vi "Teleop.vi"(10 "Match Info":T1={"Autonomous Elapsed Seconds"=0.0, "TeleOp Elapsed Seconds"=0.0, "Disabled Elapsed Seconds"=0.0, "Visited Autonomous"=FALSE, "Visited TeleOp"=FALSE, "Visited Disabled"=FALSE, "Autonomous Settings"={"Autonomous Style"=enum."Independent", "VI Refnum"=refnum}}, 11 "Call Context":T2) -> ()   [LabVIEW 2016]
doc: "This VI is called for each TeleOp packet received from the DS where the robot is not disabled. It is often used to read from the joysticks and update I/O or to update setpoints for timed control loops. It should complete and return within 20 milliseconds or it may miss DS packets."
uses:
  <vilib>/Rock Robotics/WPI/DriverStation/WPI_DriverStationDerivedRobotMode.ctl
  <vilib>/Rock Robotics/WPI/DriverStation/WPI_DriverStationMatch Info.ctl
  <vilib>/Rock Robotics/WPI/Relay/WPI_RelayValue.ctl
  <vilib>/Rock Robotics/WPI/Solenoid/WPI_SolenoidValue.ctl
  <vilib>/Rock Robotics/WPI/Utilities/WPI_GetSetVariantRefNum.vi
  <vilib>/Rock Robotics/Network Tables/NT Write Boolean Array.vi
  <vilib>/Rock Robotics/Network Tables/NT Write Numeric Array.vi
  <vilib>/Rock Robotics/Network Tables/NT Read Boolean.vi
  <vilib>/Rock Robotics/Network Tables/NT Read Number.vi
  <vilib>/Rock Robotics/WPI/RobotDrive/WPI_RobotDriveMecanumDrive_Cartesian.vi
  <vilib>/Rock Robotics/WPI/Solenoid/WPI_SolenoidSetEnum.vi
panel:
  out "Joystick Button 12":bool
  out "Joystick Button 8":bool
  in  "Test Switch 1":bool
  in  "Test Switch 3":bool
  in  "Test Switch 2":bool
  out "Ctl State 3":dbl
  out "Joystick Button 6":bool
  out "Joystick Button 4":bool
  out "Ctl State 2":dbl
  out "Joystick Button 3":bool
  out "Joystick Button 5":bool
  out "Ctl State":dbl
  out "Joystick Button 11":bool
  out "Joystick Button 7":bool
  out "Joystick Test Y":dbl
  out "Sample Slider 0":dbl(slide) scale=0.0..5.0
  out "Sample Boolean 1":bool
  out "Sample Boolean 0":bool
  # "Rope Collector"
  # "Rope Collector"
  # "Gear Arm"
  # "Gear Gripper"
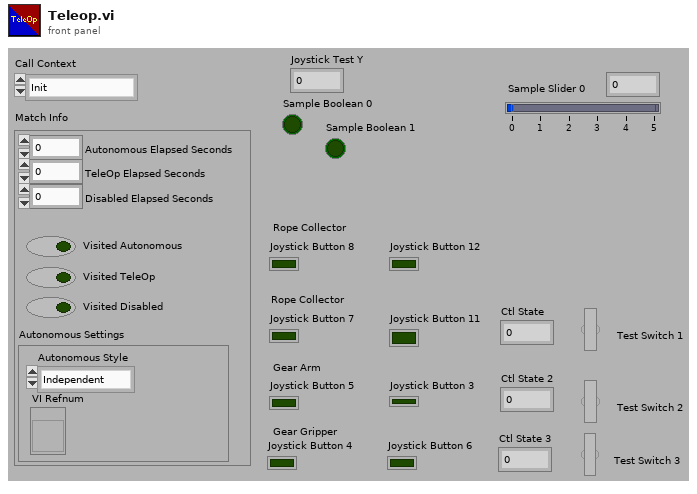
[diagram p1: front panel]
types:
  T1 = typedef "WPI_DriverStationMatch Info.ctl" = cluster{"Autonomous Elapsed Seconds":dbl, "TeleOp Elapsed Seconds":dbl, "Disabled Elapsed Seconds":dbl, "Visited Autonomous":bool, "Visited TeleOp":bool, "Visited Disabled":bool, "Autonomous Settings":cluster{"Autonomous Style":enum16{"Iterative", "Independent"}, "VI Refnum":refnum<vi>}}
  T2 = typedef "WPI_DriverStationDerivedRobotMode.ctl" = enum16{"Init", "Execute", "Stop"}
  T3 = typedef "WPI_RelayValue.ctl" = enum16{"Off", "On", "Forward", "Reverse"}
  T4 = typedef "WPI_CompressorDevRef.ctl" = cluster{"DevStatus":errorcluster, "Pneumatics Control Module":u8}
  T5 = typedef "WPI_RobotDriveDevRef.ctl" = cluster{"DevStatus":errorcluster, "Motors[]":T6[], "Square Inputs":bool, "Max Output":dbl}
  T6 = typedef "WPI_MotorControlDeviceRef.ctl" = cluster{"DeviceStatus":errorcluster, "Type":T7, "PWM":cluster{"PWM Channel":T8, "DeadBand":T9}, "CAN":cluster{"Device Number":u8, "SetOutput VI Ref":variant, "GetOutput VI Ref":variant, "Enable VI Ref":variant, "Disable VI Ref":variant, "Data":variant}, "Invert":bool}
  T7 = typedef "WPI_MotorControlType.ctl" = enum16{"PWM", "CAN"}
  T8 = typedef "FPGA_DIOPWMChannel.ctl" = enum8{"PWM 0", "PWM 1", "PWM 2", "PWM 3", "PWM 4", "PWM 5", "PWM 6", "PWM 7", "PWM 8", "PWM 9", "PWM MXP 0", "PWM MXP 1", "PWM MXP 2", "PWM MXP 3", "PWM MXP 4", "PWM MXP 5", "PWM MXP 6", "PWM MXP 7", "PWM MXP 8", "PWM MXP 9", "Invalid"}
  T9 = typedef "WPI_PWMDeadband.ctl" = cluster{"Name":string, "maxPositivePwm":i32, "minPositivePwm":i32, "centerPwm":i32, "maxNegativePwm":i32, "minNegativePwm":i32, "angularRange":u16}
  T10 = typedef "WPI_JoystickDevRef.ctl" = cluster{"Device":T11}
  T11 = typedef "WPI_JoystickDeviceEnum.ctl" = enum16{"USB 0", "USB 1", "USB 2", "USB 3", "USB 4", "USB 5"}
  T12 = cluster{"Buttons[0]":bool, "Buttons[1]":bool, "Buttons[2]":bool, "Buttons[3]":bool, "Buttons[4]":bool, "Buttons[5]":bool, "Buttons[6]":bool, "Buttons[7]":bool, "Buttons[8]":bool}
  T13 = cluster{"Axes[0]":dbl, "Axes[1]":dbl, "Axes[2]":dbl, "Axes[3]":dbl, "Axes[4]":dbl, "Axes[5]":dbl, "Axes[6]":dbl, "Axes[7]":dbl, "Axes[8]":dbl}
  T14 = typedef "WPI_RelayDevRef.ctl" = cluster{"DevStatus":errorcluster, "Relay Channel":T15, "Relay Direction":T16}
  T15 = typedef "FPGA_DIORelayChannel.ctl" = enum8{"Relay 0", "Relay 1", "Relay 2", "Relay 3", "Invalid"}
  T16 = typedef "WPI_RelayDirection.ctl" = enum16{"Both directions", "Forward only", "Reverse only"}
  T17 = typedef "WPI_SolenoidDevRef.ctl" = cluster{"DevStatus":errorcluster, "Pneumatics Control Module":u8, "Forward Solenoid Channel":T18, "Reverse Solenoid Channel":T18}
  T18 = typedef "WPI_SolenoidChannel.ctl" = enum8{"Solenoid 0", "Solenoid 1", "Solenoid 2", "Solenoid 3", "Solenoid 4", "Solenoid 5", "Solenoid 6", "Solenoid 7", "Invalid"}
  T19 = typedef "WPI_SolenoidValue.ctl" = enum16{"Off", "On", "Forward", "Reverse"}
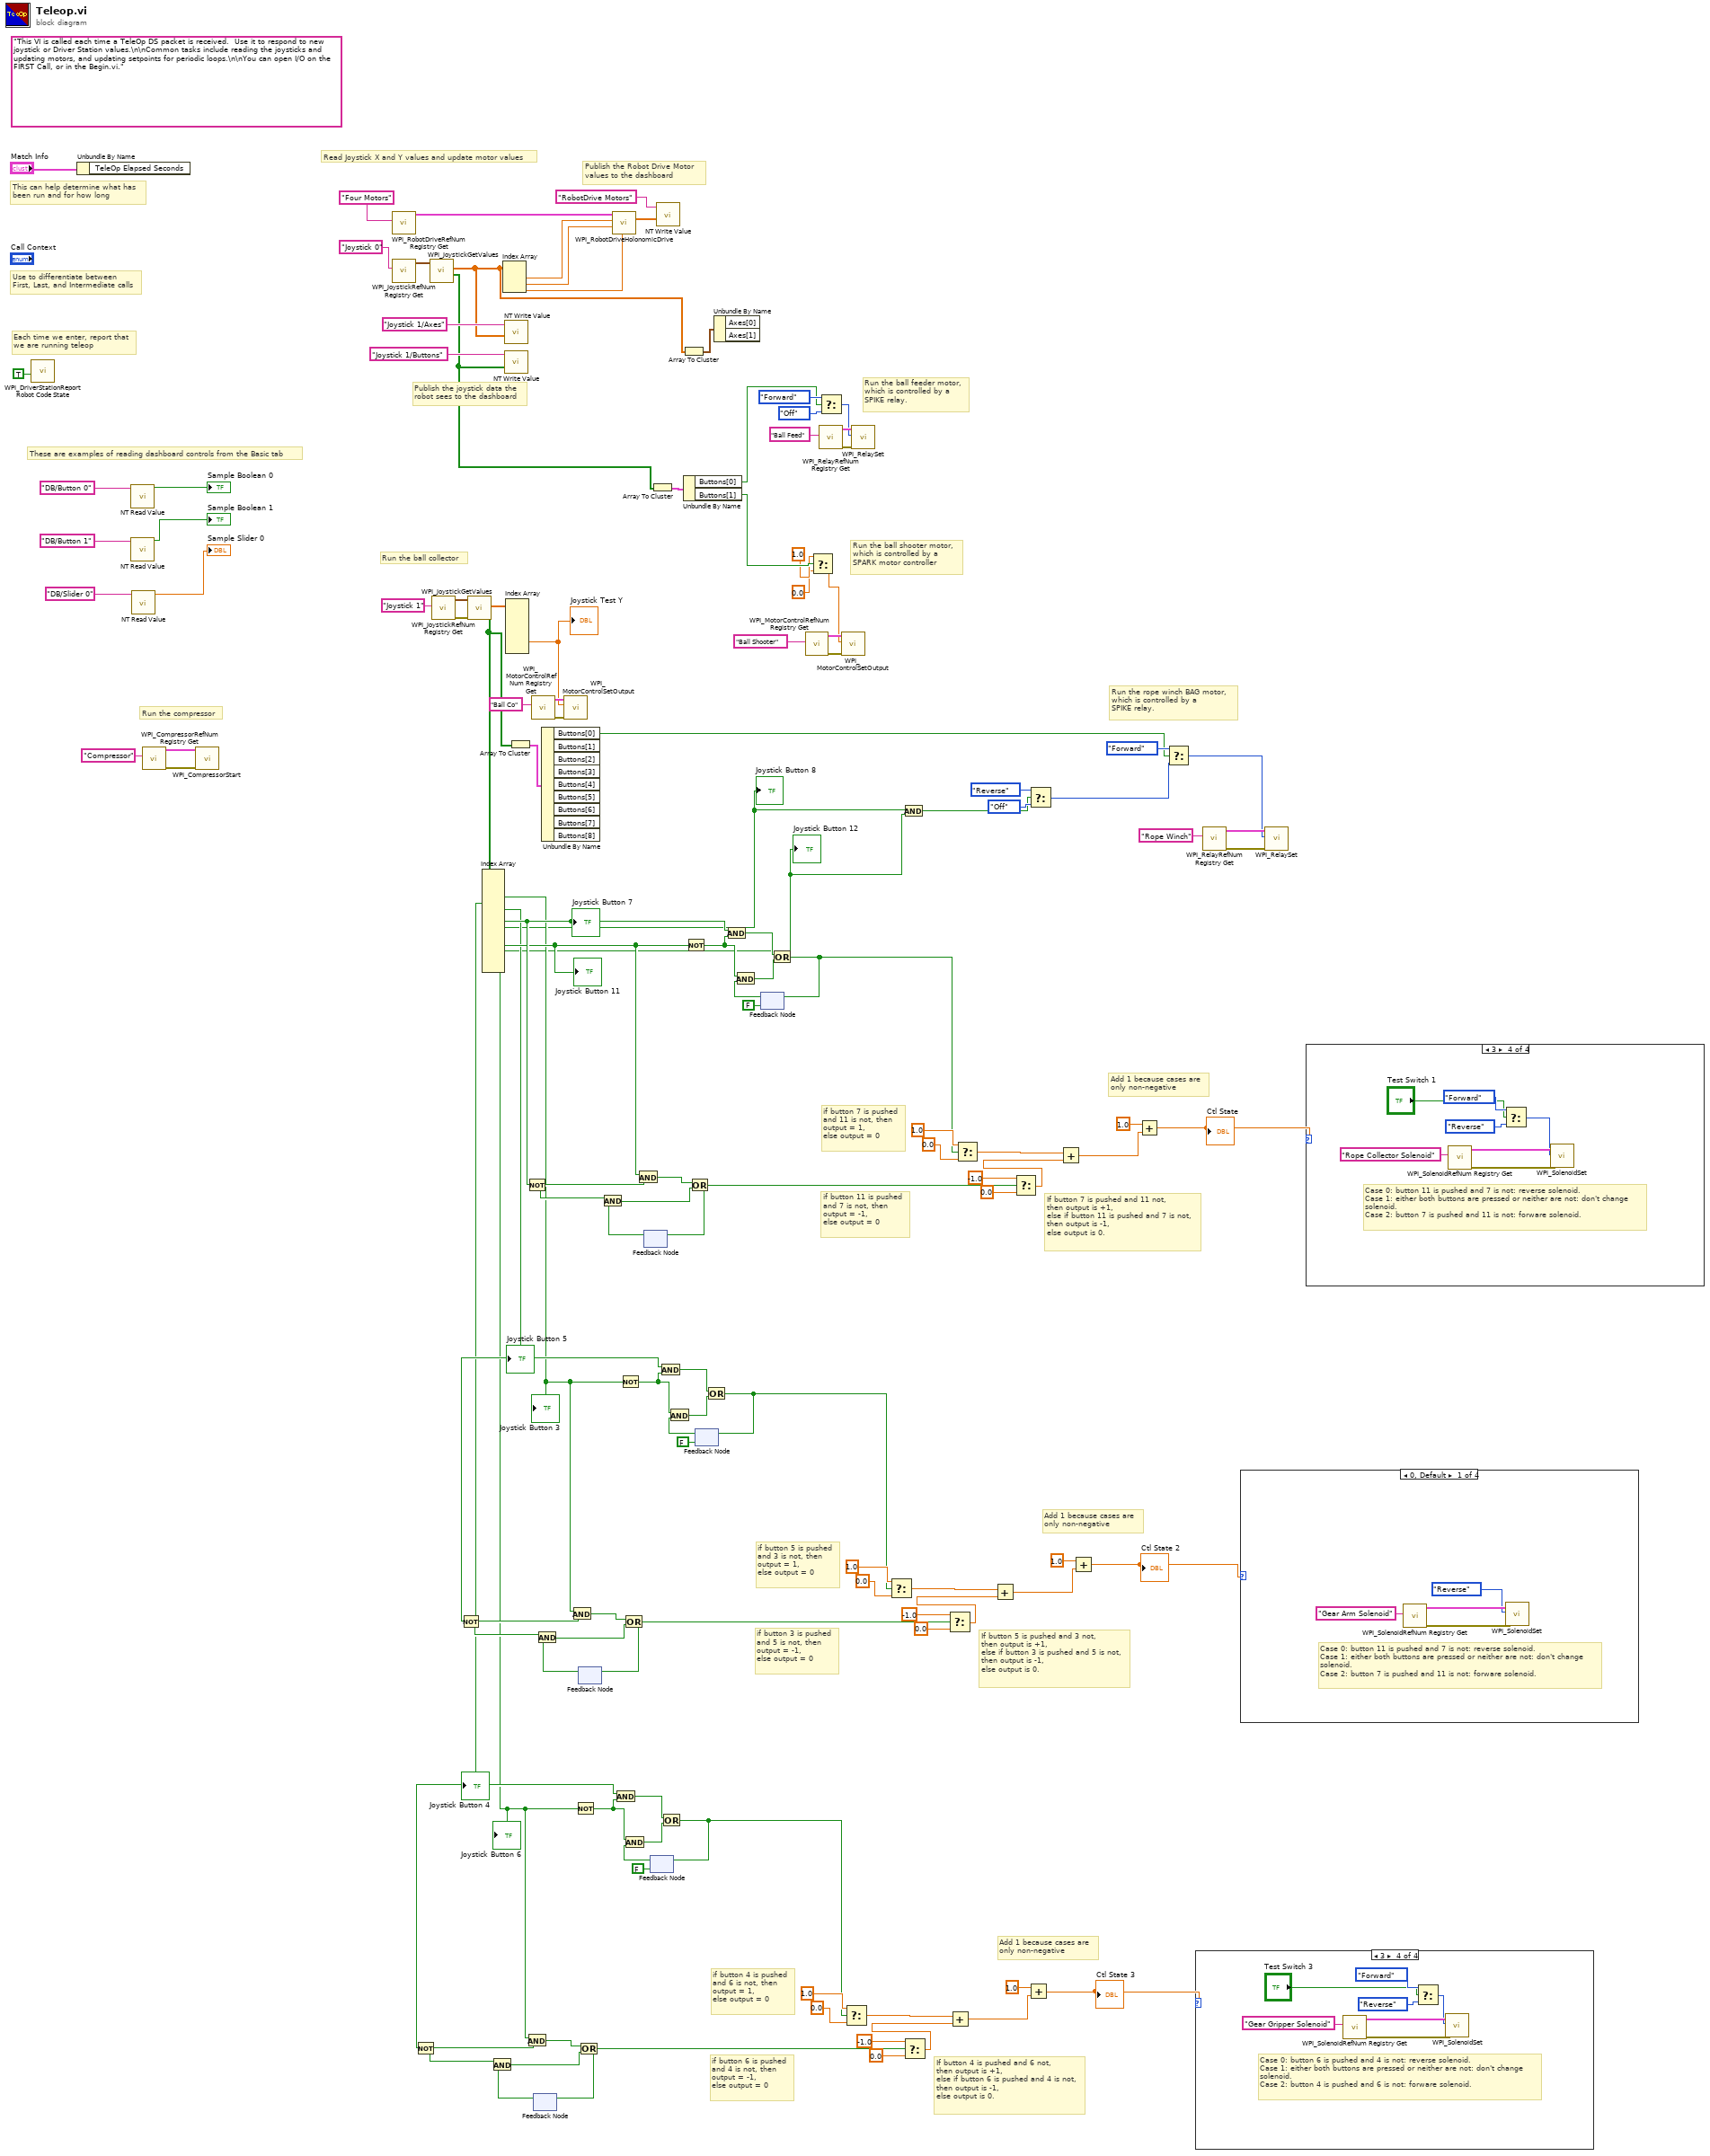
[diagram p0: block diagram]
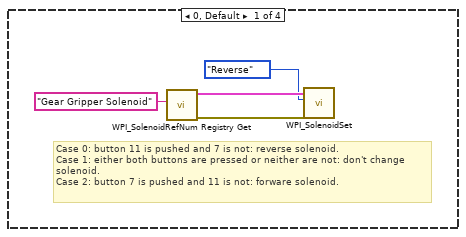
[diagram p2: hidden frame]
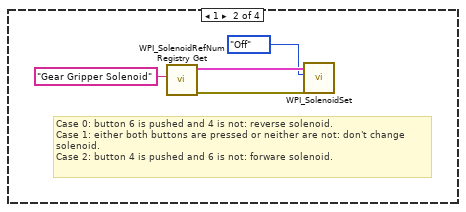
[diagram p3: hidden frame]
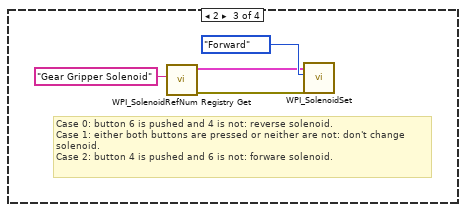
[diagram p4: hidden frame]
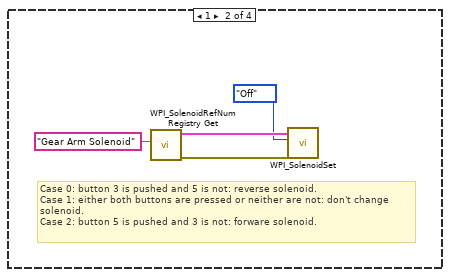
[diagram p5: hidden frame]
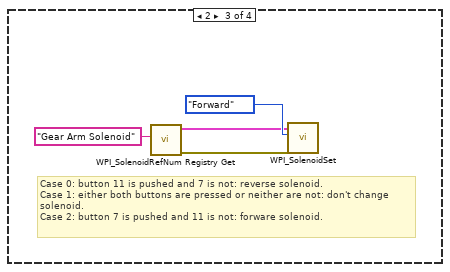
[diagram p6: hidden frame]
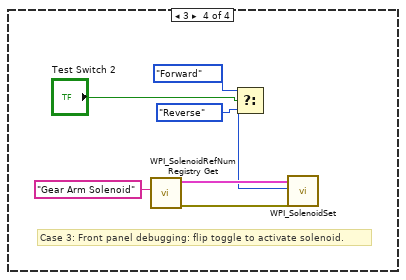
[diagram p7: hidden frame]
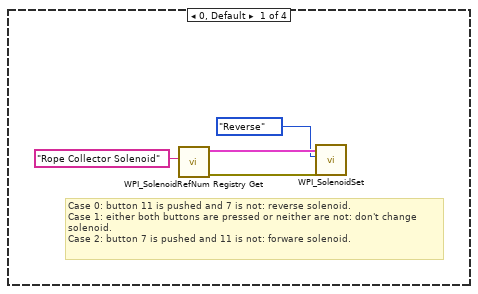
[diagram p8: hidden frame]
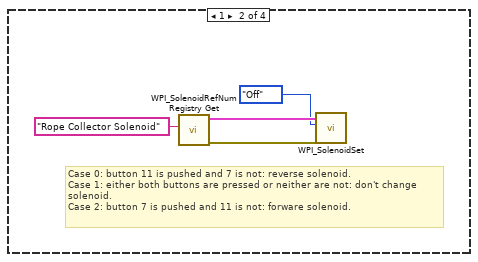
[diagram p9: hidden frame]
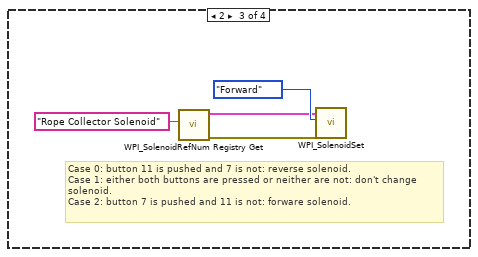
[diagram p10: hidden frame]
diagram:
  (unwired) "This VI is called each time a TeleOp DS packet is received.  Use it to respond to new joystick or Driver Station values.\n\nCommon tasks include reading the joysticks and updating motors, and updating setpoints for periodic loops.\n\nYou can open I/O on the FIRST Call, or in the Begin.vi."
  # "Add 1 because cases are \nonly non-negative"
  # "If button 4 is pushed and 6 not,\nthen output is +1,\nelse if button 6 is pushed and 4 is not,\nthen output is -1,\nelse output is 0."
  # "if button 6 is pushed\nand 4 is not, then\noutput = -1,\nelse output = 0"
  # "if button 4 is pushed\nand 6 is not, then\noutput = 1,\nelse output = 0"
  # "Add 1 because cases are \nonly non-negative"
  # "If button 5 is pushed and 3 not,\nthen output is +1,\nelse if button 3 is pushed and 5 is not,\nthen output is -1,\nelse output is 0."
  # "if button 3 is pushed\nand 5 is not, then\noutput = -1,\nelse output = 0"
  # "if button 5 is pushed\nand 3 is not, then\noutput = 1,\nelse output = 0"
  # "Add 1 because cases are \nonly non-negative"
  # "If button 7 is pushed and 11 not,\nthen output is +1,\nelse if button 11 is pushed and 7 is not,\nthen output is -1,\nelse output is 0."
  # "if button 11 is pushed\nand 7 is not, then\noutput = -1,\nelse output = 0"
  # "if button 7 is pushed\nand 11 is not, then\noutput = 1,\nelse output = 0"
  # "Run the compressor"
  # "Run the rope winch BAG motor,\nwhich is controlled by a \nSPIKE relay."
  # "Run the ball feeder motor,\nwhich is controlled by a \nSPIKE relay."
  # "Run the ball shooter motor,\nwhich is controlled by a \nSPARK motor controller"
  # "Run the ball collector"
  # "These are examples of reading dashboard controls from the Basic tab"
  # "Publish the Robot Drive Motor\nvalues to the dashboard"
  # "Publish the joystick data the\nrobot sees to the dashboard"
  # "Each time we enter, report that\nwe are running teleop"
  # "Use to differentiate between\nFirst, Last, and Intermediate calls"
  # "This can help determine what has\nbeen run and for how long"
  # "Read Joystick X and Y values and update motor values"
  n1 = call <vilib>:"WPI_DriverStationReport Robot Code State.vi"("TeleOp"=TRUE ("Autonomous")) -> ()  [unwired: 10 in, 1 out]
  n2 = Unbundle By Name("Match Info") -> ()  [unwired: 1 out]
  n3 = call-poly <vilib>:"NT Read Value.vi"("Name"="DB/Button 0" ("refnum name")) -> ("Boolean"=→"Sample Boolean 0":bool)  [unwired: 9 in, 1 out]
  n4 = call-poly <vilib>:"NT Read Value.vi"("Name"="DB/Button 1" ("refnum name")) -> ("Boolean"=→"Sample Boolean 1":bool)  [unwired: 9 in, 1 out]
  n5 = call-poly <vilib>:"NT Read Value.vi"("Name"="DB/Slider 0" ("refnum name")) -> ("Numeric"=→"Sample Slider 0":dbl)  [unwired: 9 in, 1 out]
  n6 = call <vilib>:"WPI_CompressorRefNum Registry Get.vi"("refnum name"="Compressor") -> ("error out"=w79:errorcluster, "CompressorDevRef"=w80:T4)  [unwired: 9 in]
  n7 = call <vilib>:"WPI_CompressorStart.vi"("error in (no error)"=w79, "CompressorDevRef"=w80) -> ()  [unwired: 8 in, 2 out]
  n8 = call <vilib>:"WPI_RobotDriveRefNum Registry Get.vi"("refnum name"="Four Motors") -> ("RobotDriveDevRef"=w126:T5)  [unwired: 1 in, 9 out]
  n9 = call <vilib>:"WPI_JoystickRefNum Registry Get.vi"("refnum name"="Joystick 0") -> ("JoystickDevRef"=w123:T10)  [unwired: 1 in, 9 out]
  n10 = call <vilib>:"WPI_JoystickGetValues.vi"("JoystickDevRef"=w123) -> ("Buttons"=w97:bool[], "Axes"=w98:dbl[])  [unwired: 6 in, 3 out]
  n11 = call <vilib>:"WPI_JoystickRefNum Registry Get.vi"("refnum name"="Joystick 1") -> ("error out"=w108:errorcluster, "JoystickDevRef"=w109:T10)  [unwired: 9 in]
  n12 = call <vilib>:"WPI_JoystickGetValues.vi"("error in (no error)"=w108, "JoystickDevRef"=w109) -> ("Buttons"=w8:bool[], "Axes"=w85:dbl[])  [unwired: 5 in, 3 out]
  n13 = Index Array(array=w8) -> (element #3=w18:bool, element #4=w17:bool, element #5=w19:bool, element #6=w16:bool, element #7=w78:bool, element #8=w6:bool, element #11=w60:bool, element #12=w5:bool)  [unwired: 15 in, 7 out]
  "Joystick Button 7" <- w78
  "Joystick Button 11" <- w60
  "Joystick Button 5" <- w19
  "Joystick Button 3" <- w18
  "Joystick Button 4" <- w17
  "Joystick Button 6" <- w16
  "Joystick Button 8" <- w6
  "Joystick Button 12" <- w5
  n14 = Not(x=w17) -> (.not. x?=w22:bool)
  n15 = Not(x=w19) -> (.not. x?=w41:bool)
  n16 = Index Array(array=w98) -> (element #1=w125:dbl, element #2=w120:dbl, element #3=w121:dbl)  [unwired: 3 in]
  n17 = call-poly <vilib>:"NT Write Value.vi"("Numeric Array"=w98, "Name"="Joystick 1/Axes") -> ()  [unwired: 9 in, 1 out]
  n18 = call-poly <vilib>:"NT Write Value.vi"("Boolean Array"=w97, "Name"="Joystick 1/Buttons") -> ()  [unwired: 9 in, 1 out]
  n19 = Index Array(array=w85) -> (element #2=w84:dbl)  [unwired: 7 in, 6 out]
  "Joystick Test Y" <- w84
  n20 = Array To Cluster(array=w8) -> (cluster=w89:T12)
  n21 = Not(x=w78) -> (.not. x?=w61:bool)
  n22 = And(x=w16, y=w22) -> (x .and. y?=w25:bool)
  n23 = call <vilib>:"WPI_MotorControlRefNum Registry Get.vi"("refnum name"="Ball Co") -> ("error out"=w87:errorcluster, "MotorControlDevRef"=w88:T6)  [unwired: 9 in]
  n24 = feedback #1() -> (w23:bool)  [unwired: 1 in]
  n25 = And(x=w22, y=w23) -> (x .and. y?=w24:bool)
  n26 = Unbundle By Name(w89) -> ("Buttons[0]"=w12:bool)  [unwired: 8 out]
  n27 = call <vilib>:"WPI_MotorControlSetOutput.vi"("error in (no error)"=w87, "Output"=w84, "MotorControlDevRef"=w88) -> ()  [unwired: 6 in, 3 out]
  n28 = And(x=w18, y=w41) -> (x .and. y?=w44:bool)
  n29 = Not(x=w16) -> (.not. x?=w31:bool)
  n30 = Or(x=w25, y=w24) -> (x .or. y?=w21:bool)
  n31 = feedback-in #1(w21) -> ()
  n32 = feedback #2() -> (w42:bool)  [unwired: 1 in]
  n33 = And(x=w41, y=w42) -> (x .and. y?=w43:bool)
  n34 = call-poly <vilib>:"WPI_RobotDriveHolonomicDrive.vi"("Rotation"=w121, "Y"=w120, "X"=w125, "RobotDriveDevRef"=w126) -> ("Motor Values"=w117:dbl[])  [unwired: 5 in, 2 out]
  n35 = And(x=w17, y=w31) -> (x .and. y?=w30:bool)
  n36 = Not(x=w18) -> (.not. x?=w50:bool)
  n37 = Or(x=w44, y=w43) -> (x .or. y?=w40:bool)
  n38 = feedback-in #2(w40) -> ()
  n39 = And(x=w60, y=w61) -> (x .and. y?=w64:bool)
  n40 = feedback #3() -> (w62:bool)  [unwired: 1 in]
  n41 = And(x=w61, y=w62) -> (x .and. y?=w63:bool)
  n42 = feedback #4(FALSE) -> (w28:bool)
  n43 = And(x=w31, y=w28) -> (x .and. y?=w29:bool)
  n44 = Array To Cluster(array=w97) -> (cluster=w107:T12)
  n45 = call-poly <vilib>:"NT Write Value.vi"("Numeric Array"=w117, "Name"="RobotDrive Motors") -> ()  [unwired: 9 in, 1 out]
  n46 = And(x=w19, y=w50) -> (x .and. y?=w49:bool)
  n47 = Or(x=w30, y=w29) -> (x .or. y?=w26:bool)
  n48 = feedback-in #4(w26) -> ()
  n49 = Array To Cluster(array=w98) -> (cluster=w106:T13)
  n50 = Unbundle By Name(w107) -> ("Buttons[0]"=w92:bool, "Buttons[1]"=w102:bool)
  n51 = Not(x=w60) -> (.not. x?=w70:bool)
  n52 = Or(x=w64, y=w63) -> (x .or. y?=w59:bool)
  n53 = feedback-in #3(w59) -> ()
  n54 = feedback #5(FALSE) -> (w47:bool)
  n55 = And(x=w50, y=w47) -> (x .and. y?=w48:bool)
  n56 = Or(x=w49, y=w48) -> (x .or. y?=w45:bool)
  n57 = feedback-in #5(w45) -> ()
  n58 = Unbundle By Name(w106) -> ()  [unwired: 2 out]
  n59 = And(x=w78, y=w70) -> (x .and. y?=w69:bool)
  n60 = feedback #6(FALSE) -> (w67:bool)
  n61 = And(x=w70, y=w67) -> (x .and. y?=w68:bool)
  n62 = Or(x=w69, y=w68) -> (x .or. y?=w65:bool)
  n63 = feedback-in #6(w65) -> ()
  n64 = call <vilib>:"WPI_MotorControlRefNum Registry Get.vi"("refnum name"="Ball Shooter") -> ("error out"=w103:errorcluster, "MotorControlDevRef"=w104:T6)  [unwired: 9 in]
  n65 = Select(t=1.0, s=w102, f=0.0) -> (s? t:f=w99:dbl)
  n66 = Select(t=WPI_RelayValue."Forward" ("RelayValue"), s=w92, f=WPI_RelayValue."Off" ("RelayValue")) -> (s? t:f=w90:T3)
  n67 = call <vilib>:"WPI_RelayRefNum Registry Get.vi"("refnum name"="Ball Feed") -> ("error out"=w95:errorcluster, "RelayDevRef"=w96:T14)  [unwired: 9 in]
  n68 = call <vilib>:"WPI_MotorControlSetOutput.vi"("error in (no error)"=w103, "Output"=w99, "MotorControlDevRef"=w104) -> ()  [unwired: 6 in, 3 out]
  n69 = Select(t=1.0, s=w26, f=0.0) -> (s? t:f=w36:dbl)
  n70 = call <vilib>:"WPI_RelaySet.vi"("error in (no error)"=w95, "RelayValue"=w90, "RelayDevRef"=w96) -> ()  [unwired: 7 in, 2 out]
  n71 = Select(t=1.0, s=w45, f=0.0) -> (s? t:f=w55:dbl)
  n72 = And(x=w6, y=w5) -> (x .and. y?=w1:bool)
  n73 = Select(t=-1.0, s=w21, f=0.0) -> (s? t:f=w37:dbl)
  n74 = Select(t=-1.0, s=w40, f=0.0) -> (s? t:f=w56:dbl)
  n75 = Add(x=w36, y=w37) -> (x+y=w38:dbl)
  n76 = Select(t=1.0, s=w65, f=0.0) -> (s? t:f=w75:dbl)
  n77 = Add(x=w55, y=w56) -> (x+y=w57:dbl)
  n78 = Select(t=-1.0, s=w59, f=0.0) -> (s? t:f=w76:dbl)
  n79 = Add(x=1.0, y=w38) -> (x+y=w13:dbl)
  "Ctl State 3" <- w13
  n80 = Select(t=WPI_RelayValue."Reverse" ("RelayValue"), s=w1, f=WPI_RelayValue."Off" ("RelayValue")) -> (s? t:f=w2:T3)
  n81 = Add(x=w75, y=w76) -> (x+y=w77:dbl)
  n82 = Add(x=1.0, y=w57) -> (x+y=w14:dbl)
  "Ctl State 2" <- w14
  n83 = Add(x=1.0, y=w77) -> (x+y=w15:dbl)
  "Ctl State" <- w15
  n84 = Select(t=WPI_RelayValue."Forward" ("RelayValue"), s=w12, f=w2) -> (s? t:f=w7:T3)
  n85 = case shown="3" w13 {
    frame 0, Default {
      # "Case 0: button 11 is pushed and 7 is not: reverse solenoid.\nCase 1: either both buttons are pressed or neither are not: don't change\nsolenoid.\nCase 2: button 7 is pushed and 11 is not: forware solenoid."
      n86 = call <vilib>:"WPI_SolenoidRefNum Registry Get.vi"("refnum name"="Gear Gripper Solenoid") -> ("error out"=w132:errorcluster, "SolenoidDevRef"=w131:T17)  [unwired: 9 in]
      n87 = call-poly <vilib>:"WPI_SolenoidSet.vi"("error in (no error)"=w132, "Value"=WPI_RelayValue."Reverse" ("RelayValue"), "SolenoidDevRef"=w131) -> ()  [unwired: 7 in, 2 out]
    }
    frame 1 {
      # "Case 0: button 6 is pushed and 4 is not: reverse solenoid.\nCase 1: either both buttons are pressed or neither are not: don't change\nsolenoid.\nCase 2: button 4 is pushed and 6 is not: forware solenoid."
      n88 = call <vilib>:"WPI_SolenoidRefNum Registry Get.vi"("refnum name"="Gear Gripper Solenoid") -> ("error out"=w136:errorcluster, "SolenoidDevRef"=w135:T17)  [unwired: 9 in]
      n89 = call-poly <vilib>:"WPI_SolenoidSet.vi"("error in (no error)"=w136, "Value"=WPI_RelayValue."Off" ("RelayValue"), "SolenoidDevRef"=w135) -> ()  [unwired: 7 in, 2 out]
    }
    frame 2 {
      # "Case 0: button 6 is pushed and 4 is not: reverse solenoid.\nCase 1: either both buttons are pressed or neither are not: don't change\nsolenoid.\nCase 2: button 4 is pushed and 6 is not: forware solenoid."
      n90 = call <vilib>:"WPI_SolenoidRefNum Registry Get.vi"("refnum name"="Gear Gripper Solenoid") -> ("error out"=w137:errorcluster, "SolenoidDevRef"=w138:T17)  [unwired: 9 in]
      n91 = call-poly <vilib>:"WPI_SolenoidSet.vi"("error in (no error)"=w137, "Value"=WPI_RelayValue."Forward" ("RelayValue"), "SolenoidDevRef"=w138) -> ()  [unwired: 7 in, 2 out]
    }
    frame 3 {
      # "Case 0: button 6 is pushed and 4 is not: reverse solenoid.\nCase 1: either both buttons are pressed or neither are not: don't change\nsolenoid.\nCase 2: button 4 is pushed and 6 is not: forware solenoid."
      n92 = call <vilib>:"WPI_SolenoidRefNum Registry Get.vi"("refnum name"="Gear Gripper Solenoid") -> ("error out"=w147:errorcluster, "SolenoidDevRef"=w146:T17)  [unwired: 9 in]
      n93 = Select(t=WPI_RelayValue."Forward" ("RelayValue"), s="Test Switch 3", f=WPI_RelayValue."Reverse" ("RelayValue")) -> (s? t:f=w141:T3)
      n94 = call-poly <vilib>:"WPI_SolenoidSet.vi"("error in (no error)"=w147, "Value"=w141, "SolenoidDevRef"=w146) -> ()  [unwired: 7 in, 2 out]
    }
  }
  n95 = call <vilib>:"WPI_RelayRefNum Registry Get.vi"("refnum name"="Rope Winch") -> ("error out"=w10:errorcluster, "RelayDevRef"=w11:T14)  [unwired: 9 in]
  n96 = case shown="0, Default" w14 {
    frame 0, Default {
      # "Case 0: button 11 is pushed and 7 is not: reverse solenoid.\nCase 1: either both buttons are pressed or neither are not: don't change\nsolenoid.\nCase 2: button 7 is pushed and 11 is not: forware solenoid."
      n97 = call <vilib>:"WPI_SolenoidRefNum Registry Get.vi"("refnum name"="Gear Arm Solenoid") -> ("error out"=w151:errorcluster, "SolenoidDevRef"=w150:T17)  [unwired: 9 in]
      n98 = call-poly <vilib>:"WPI_SolenoidSet.vi"("error in (no error)"=w151, "Value"=WPI_RelayValue."Reverse" ("RelayValue"), "SolenoidDevRef"=w150) -> ()  [unwired: 7 in, 2 out]
    }
    frame 1 {
      # "Case 0: button 3 is pushed and 5 is not: reverse solenoid.\nCase 1: either both buttons are pressed or neither are not: don't change\nsolenoid.\nCase 2: button 5 is pushed and 3 is not: forware solenoid."
      n99 = call <vilib>:"WPI_SolenoidRefNum Registry Get.vi"("refnum name"="Gear Arm Solenoid") -> ("error out"=w155:errorcluster, "SolenoidDevRef"=w154:T17)  [unwired: 9 in]
      n100 = call-poly <vilib>:"WPI_SolenoidSet.vi"("error in (no error)"=w155, "Value"=WPI_SolenoidValue."Off", "SolenoidDevRef"=w154) -> ()  [unwired: 7 in, 2 out]
    }
    frame 2 {
      # "Case 0: button 11 is pushed and 7 is not: reverse solenoid.\nCase 1: either both buttons are pressed or neither are not: don't change\nsolenoid.\nCase 2: button 7 is pushed and 11 is not: forware solenoid."
      n101 = call <vilib>:"WPI_SolenoidRefNum Registry Get.vi"("refnum name"="Gear Arm Solenoid") -> ("error out"=w156:errorcluster, "SolenoidDevRef"=w157:T17)  [unwired: 9 in]
      n102 = call-poly <vilib>:"WPI_SolenoidSet.vi"("error in (no error)"=w156, "Value"=WPI_RelayValue."Forward" ("RelayValue"), "SolenoidDevRef"=w157) -> ()  [unwired: 7 in, 2 out]
    }
    frame 3 {
      # "Case 3: Front panel debugging: flip toggle to activate solenoid."
      n103 = call <vilib>:"WPI_SolenoidRefNum Registry Get.vi"("refnum name"="Gear Arm Solenoid") -> ("error out"=w166:errorcluster, "SolenoidDevRef"=w165:T17)  [unwired: 9 in]
      n104 = Select(t=WPI_RelayValue."Forward" ("RelayValue"), s="Test Switch 2", f=WPI_RelayValue."Reverse" ("RelayValue")) -> (s? t:f=w160:T3)
      n105 = call-poly <vilib>:"WPI_SolenoidSet.vi"("error in (no error)"=w166, "Value"=w160, "SolenoidDevRef"=w165) -> ()  [unwired: 7 in, 2 out]
    }
  }
  n106 = call <vilib>:"WPI_RelaySet.vi"("error in (no error)"=w10, "RelayValue"=w7, "RelayDevRef"=w11) -> ()  [unwired: 7 in, 2 out]
  n107 = case shown="3" w15 {
    frame 0, Default {
      # "Case 0: button 11 is pushed and 7 is not: reverse solenoid.\nCase 1: either both buttons are pressed or neither are not: don't change\nsolenoid.\nCase 2: button 7 is pushed and 11 is not: forware solenoid."
      n108 = call <vilib>:"WPI_SolenoidRefNum Registry Get.vi"("refnum name"="Rope Collector Solenoid") -> ("error out"=w170:errorcluster, "SolenoidDevRef"=w169:T17)  [unwired: 9 in]
      n109 = call-poly <vilib>:"WPI_SolenoidSet.vi"("error in (no error)"=w170, "Value"=WPI_RelayValue."Reverse" ("RelayValue"), "SolenoidDevRef"=w169) -> ()  [unwired: 7 in, 2 out]
    }
    frame 1 {
      # "Case 0: button 11 is pushed and 7 is not: reverse solenoid.\nCase 1: either both buttons are pressed or neither are not: don't change\nsolenoid.\nCase 2: button 7 is pushed and 11 is not: forware solenoid."
      n110 = call <vilib>:"WPI_SolenoidRefNum Registry Get.vi"("refnum name"="Rope Collector Solenoid") -> ("error out"=w174:errorcluster, "SolenoidDevRef"=w173:T17)  [unwired: 9 in]
      n111 = call-poly <vilib>:"WPI_SolenoidSet.vi"("error in (no error)"=w174, "Value"=WPI_RelayValue."Off" ("RelayValue"), "SolenoidDevRef"=w173) -> ()  [unwired: 7 in, 2 out]
    }
    frame 2 {
      # "Case 0: button 11 is pushed and 7 is not: reverse solenoid.\nCase 1: either both buttons are pressed or neither are not: don't change\nsolenoid.\nCase 2: button 7 is pushed and 11 is not: forware solenoid."
      n112 = call <vilib>:"WPI_SolenoidRefNum Registry Get.vi"("refnum name"="Rope Collector Solenoid") -> ("error out"=w175:errorcluster, "SolenoidDevRef"=w176:T17)  [unwired: 9 in]
      n113 = call-poly <vilib>:"WPI_SolenoidSet.vi"("error in (no error)"=w175, "Value"=WPI_RelayValue."Forward" ("RelayValue"), "SolenoidDevRef"=w176) -> ()  [unwired: 7 in, 2 out]
    }
    frame 3 {
      # "Case 0: button 11 is pushed and 7 is not: reverse solenoid.\nCase 1: either both buttons are pressed or neither are not: don't change\nsolenoid.\nCase 2: button 7 is pushed and 11 is not: forware solenoid."
      n114 = call <vilib>:"WPI_SolenoidRefNum Registry Get.vi"("refnum name"="Rope Collector Solenoid") -> ("error out"=w185:errorcluster, "SolenoidDevRef"=w184:T17)  [unwired: 9 in]
      n115 = Select(t=WPI_RelayValue."Forward" ("RelayValue"), s="Test Switch 1", f=WPI_RelayValue."Reverse" ("RelayValue")) -> (s? t:f=w180:T3)
      n116 = call-poly <vilib>:"WPI_SolenoidSet.vi"("error in (no error)"=w185, "Value"=w180, "SolenoidDevRef"=w184) -> ()  [unwired: 7 in, 2 out]
    }
  }
